vi "XIPIN_AXI_Register_Slice_2_1.vi"   [LabVIEW 2017]
doc: "The AXI Register Slice IP provides the facility to add a back pressure aware pipeline between an AXI4/AXI3/AXI4-Lite master and slave.\n------------------------------------\n<b>Need License</b> : No\n<b>Interface</b> : AXI4"
uses:
  <vilib>/rvi/XilinxIP/XIPIN_XNode/niFpgaXIPIN.xnode
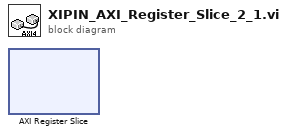
[diagram p0: block diagram]
diagram:
  n1 = xnode ("AXI Register Slice")() -> ()
